vi "TDS 2004B Three Channel Initialize SubVI 03.vi"(0 "VISA Refnum in":refnum<visa-resource-name>, 1 "Probe Attenuation Ch A":dbl, 2 "Probe Attenuation Ch B":dbl, 3 "Trigger Source":u16, 4 "Channel B":u16, 5 "Vertical Range Ch B (V/Div)":dbl, 6 "Vertical Offset Ch B (V)":dbl, 7 "error in":errorcluster, 8 "Vertical Coupling":u16, 9 "Trigger Level (-4.4 V) in":dbl, 10 "Vertical Range Ch A (V/Div)":dbl, 11 "Trigger Mode":u16, 12 "Vertical Offset Ch A (V)":dbl, 13 "Trigger Slope":i32, 14 "Channel A":u16, 15 "Timebase":dbl=0.01 format="%#_13g", 16 "Serial Configuration 3":T1, 17 "Number of Averaged Waveforms (4: 4)":i32(ring)=128 items=["4"=4, "16"=16, "64"=64, "128"=128], 19 "Acquisition Type (0: Sample)":i32(ring)=1 items=["Sample", "Average", "Peak Detect"]) -> (18 "Array":u16[](array[numeric]), 20 "VISA Refnum out":refnum<visa-resource-name>, 21 "Timeout (ms)":u32, 27 "error out":errorcluster)   [LabVIEW 2017]
uses:
  <instrlib>/Tektronix TDS 200 1000 2000 Series/Public/Configure/Configure Trigger (Edge).vi
  <instrlib>/Tektronix TDS 200 1000 2000 Series/Tektronix TDS 200 1000 2000 Series.lvlib
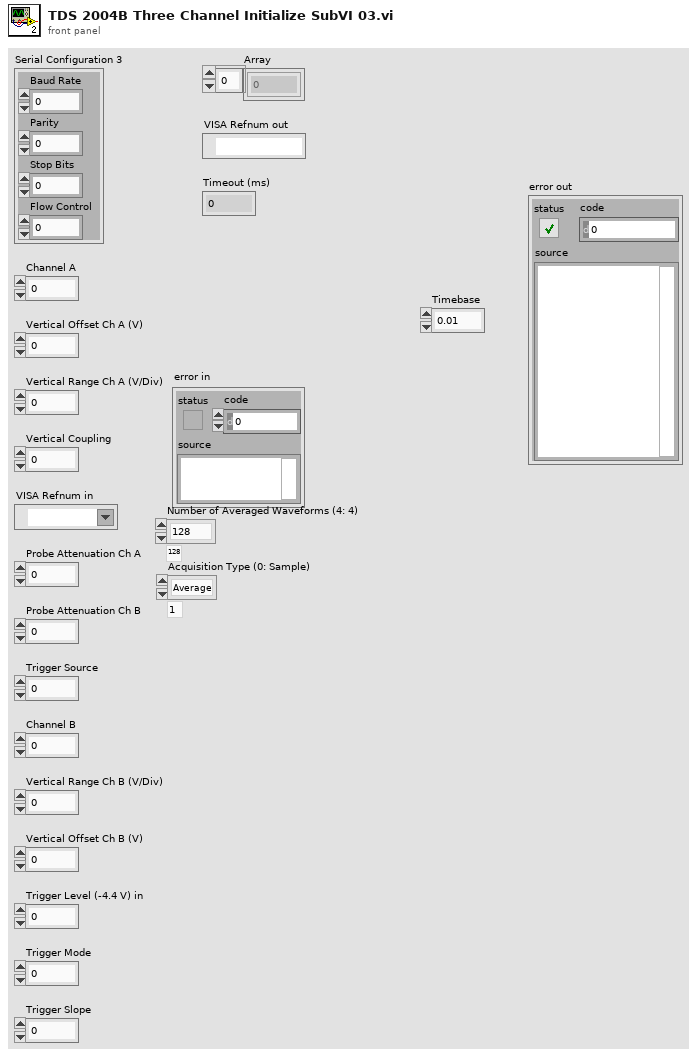
[diagram p1: front panel]
types:
  T1 = cluster{"Baud Rate":u32, "Parity":u16, "Stop Bits":u16, "Flow Control":u16}
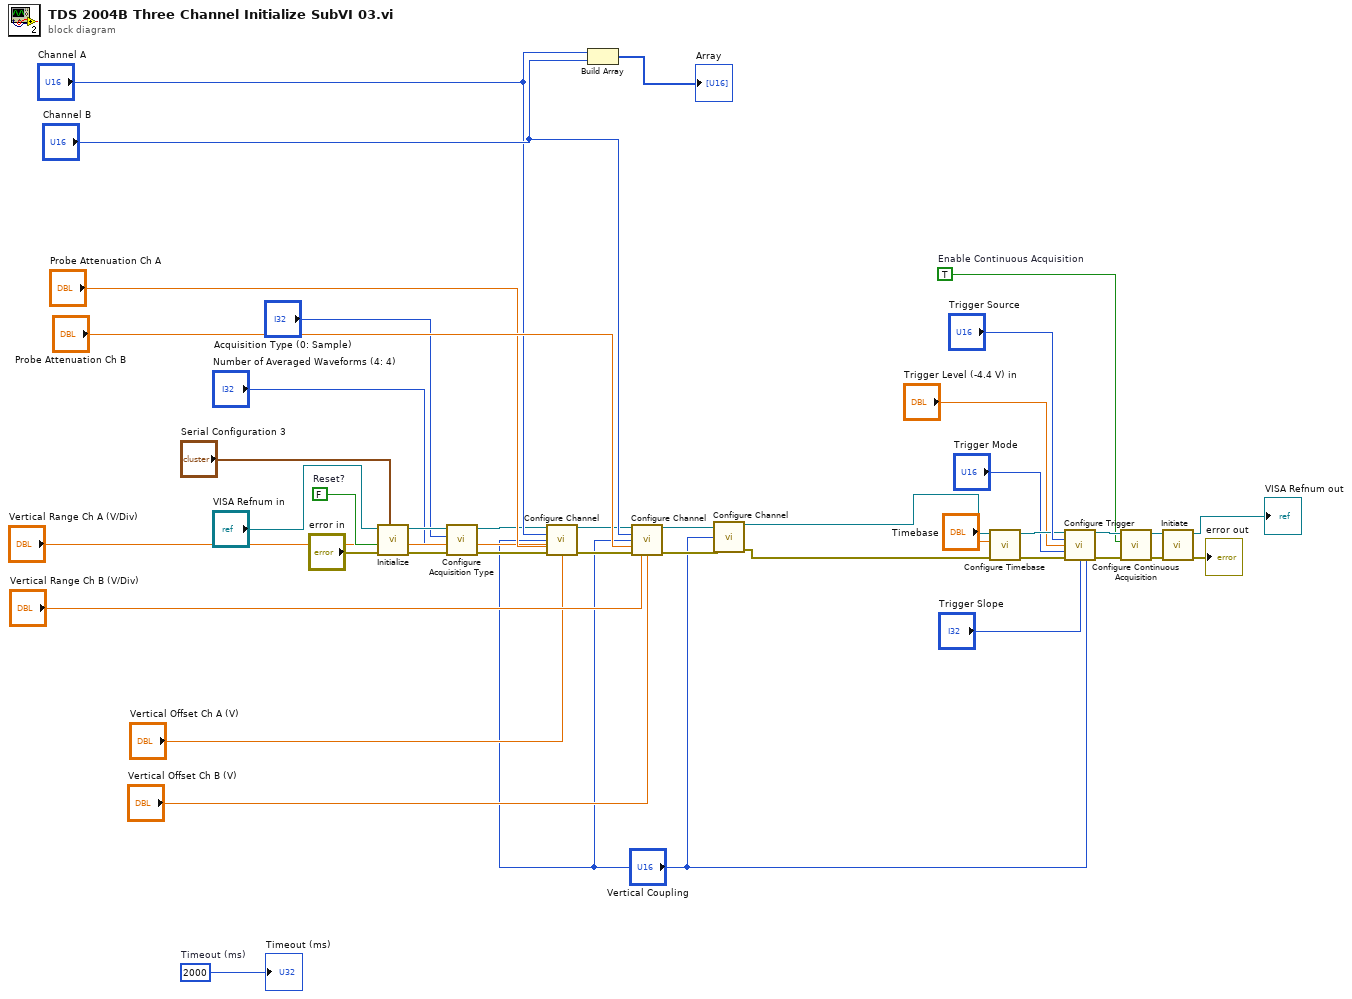
[diagram p0: block diagram]
diagram:
  w19 = FALSE  # Reset?
  w28 = u32 2000  # Timeout (ms)
  w15 = TRUE  # Enable Continuous Acquisition
  n1 = call <instrlib>:"Initialize.vi"("Serial Configuration"="Serial Configuration 3", "error in (no error)"="error in", "Reset? (T: Yes)"=w19, "VISA resource name"="VISA Refnum in") -> ("error out"=w11:errorcluster, "VISA resource name out"=w9:refnum<visa-resource-name>)  [unwired: 6 in]
  n2 = call <instrlib>:"Configure Acquisition Type.vi"("error in (no error)"=w11, "Number of Averaged Waveforms (4: 4)"="Number of Averaged Waveforms (4: 4)", "Acquisition Type (0: Sample)"="Acquisition Type (0: Sample)", "VISA resource name"=w9) -> ("error out"=w10:errorcluster, "VISA resource name out"=w8:refnum<visa-resource-name>)  [unwired: 6 in]
  n3 = call <instrlib>:"Configure Channel.vi"("VISA resource name"=w8, "Channel (0: Channel 1)"="Channel A", "Vertical Coupling (1: DC)"="Vertical Coupling", "Probe Attenuation (10: 10X)"="Probe Attenuation Ch A", "error in (no error)"=w10, "Vertical Range (10.0 V/div)"="Vertical Range Ch A (V/Div)", "Vertical Offset (0.0 divs)"="Vertical Offset Ch A (V)") -> ("VISA resource name out"=w33:refnum<visa-resource-name>, "error out"=w36:errorcluster)  [unwired: 7 in]
  n4 = Build Array("Channel A", "Channel B") -> (→"Array":u16[])
  n5 = call <instrlib>:"Configure Channel.vi"("VISA resource name"=w33, "Channel (0: Channel 1)"="Channel B", "Vertical Coupling (1: DC)"="Vertical Coupling", "Probe Attenuation (10: 10X)"="Probe Attenuation Ch B", "error in (no error)"=w36, "Vertical Range (10.0 V/div)"="Vertical Range Ch B (V/Div)", "Vertical Offset (0.0 divs)"="Vertical Offset Ch B (V)") -> ("VISA resource name out"=w5:refnum<visa-resource-name>, "error out"=w4:errorcluster)  [unwired: 7 in]
  n6 = call <instrlib>:"Configure Channel.vi"("VISA resource name"=w5, "Vertical Coupling (1: DC)"="Vertical Coupling", "error in (no error)"=w4) -> ("VISA resource name out"=w3:refnum<visa-resource-name>, "error out"=w2:errorcluster)  [unwired: 11 in]
  n7 = call <instrlib>:"Configure Timebase.vi"("error in (no error)"=w2, "Timebase (0.0005 s)"="Timebase", "VISA resource name"=w3) -> ("error out"=w22:errorcluster, "VISA resource name out"=w21:refnum<visa-resource-name>)  [unwired: 7 in]
  n8 = call-poly <instrlib>:"Configure Trigger.vi"("VISA resource name"=w21, "Trigger Source (0: Channel 1)"="Trigger Source", "Trigger Level (0.0 V)"="Trigger Level (-4.4 V) in", "Trigger Mode (0: Auto)"="Trigger Mode", "error in (no error)"=w22, "Trigger Slope (0: Rising)"="Trigger Slope", "Trigger Coupling (0: AC)"="Vertical Coupling") -> ("VISA resource name out"=w23:refnum<visa-resource-name>, "error out"=w24:errorcluster)  [unwired: 7 in]
  n9 = call <instrlib>:"Configure Continuous Acquisition.vi"("error in (no error)"=w24, "Enable Continuous Acquisition Mode (True)"=w15, "VISA resource name"=w23) -> ("error out"=w27:errorcluster, "VISA resource name out"=w25:refnum<visa-resource-name>)  [unwired: 7 in]
  n10 = call <instrlib>:"Initiate.vi"("error in (no error)"=w27, "VISA resource name"=w25) -> ("error out"=→"error out":errorcluster, "VISA resource name out"=→"VISA Refnum out":refnum<visa-resource-name>)  [unwired: 8 out]
  "Timeout (ms)" <- w28
